vi "SWERVE_DRIVE_ACT.vi"(6 "Pass_Through_Time":dbl=-1.0 format="%33.4f", 8 "in Swerve Module States":T4[](array[typedef]) {"Angle"."SIN" format="%13.4f"; "Angle"."COS" format="%13.4f"; "Angle"."VALUE" format="%13.4f"}, 9 "Gyro_Heading_Rad":dbl, 10 "Swerve Drive Device Reference":T6[](array[typedef]), 11 "in SWERVE_DRIVE_KINEMATICS":T1 {"SavedModuleStates"."Angle"."SIN" format="%13.4f"; "SavedModuleStates"."Angle"."COS" format="%13.4f"; "SavedModuleStates"."Angle"."VALUE" format="%13.4f"; "PrevCoR"."Y" format="%14.3f"; "PrevCoR"."X" format="%14.3f"; "Modules"."Y" format="%14.3f"; "Modules"."X" format="%14.3f"}) -> (3 "out SWERVE_DRIVE_KINEMATICS":T1 {"SavedModuleStates"."Angle"."SIN" format="%13.4f"; "SavedModuleStates"."Angle"."COS" format="%13.4f"; "SavedModuleStates"."Angle"."VALUE" format="%13.4f"; "PrevCoR"."Y" format="%14.3f"; "PrevCoR"."X" format="%14.3f"; "Modules"."Y" format="%14.3f"; "Modules"."X" format="%14.3f"})   [LabVIEW 2019]
uses:
  <vilib>/Rock Robotics/WPI/ThirdParty/JAS_Junk/TrajLib/TypeDef/SWERVE_DRIVE_KINEMATICS.ctl
  <vilib>/Analysis/Matrix/Datatypes/RealMatrix.ctl
  <vilib>/Rock Robotics/WPI/ThirdParty/JAS_Junk/TrajLib/TypeDef/TRANSLATION2D.ctl
  <vilib>/Rock Robotics/WPI/ThirdParty/JAS_Junk/TrajLib/TypeDef/SWERVE_DRIVE_MODULE_STATE.ctl
  <vilib>/Rock Robotics/WPI/ThirdParty/JAS_Junk/TrajLib/TypeDef/ROTATION2D.ctl
  SWERVE_DRIVE_MODULE_TYPDEF.ctl
  <vilib>/Rock Robotics/WPI/MotorControl/WPI_MotorControlDeviceRef.ctl
  <vilib>/Rock Robotics/WPI/MotorControl/WPI_MotorControlType.ctl
  <vilib>/Rock Robotics/SystemInterfaces/DIO/FPGA_DIOPWMChannel.ctl
  <vilib>/Rock Robotics/WPI/PWM/WPI_PWMDeadband.ctl
  <vilib>/Rock Robotics/SystemInterfaces/DIO/FPGA_DIOChannel.ctl
  <vilib>/Rock Robotics/WPI/Encoder/WPI_EncoderDevRef.ctl
  <vilib>/Rock Robotics/SystemInterfaces/Encoder/FPGA_EncoderIdx.ctl
  <vilib>/Rock Robotics/SystemInterfaces/Counter/FPGA_CounterCtrSystemIndex.ctl
  <vilib>/Rock Robotics/WPI/Encoder/WPI_EncoderType.ctl
  <vilib>/Rock Robotics/WPI/ThirdParty/JAS_Junk/TrajLib/TypeDef/X_Y_PAIR.ctl
  <vilib>/Rock Robotics/WPI/ThirdParty/JAS_Junk/TrajLib/VI/Util_GetTime_U32.vi
  <vilib>/Rock Robotics/WPI/ThirdParty/JAS_Junk/TrajLib/MathUtil_InputModulus.vi
  <vilib>/Rock Robotics/WPI/ThirdParty/JAS_Junk/TrajLib/VI/FunctionGenerator_New.vi
  <vilib>/Rock Robotics/WPI/ThirdParty/JAS_Junk/TrajLib/VI/FunctionGenerator_Calculate.vi
  <vilib>/Rock Robotics/WPI/ThirdParty/JAS_Junk/TrajLib/PIDController_AtSetpoint.vi
  <vilib>/Rock Robotics/WPI/ThirdParty/JAS_Junk/TrajLib/PIDController_SetPIDF.vi
  <vilib>/Rock Robotics/WPI/ThirdParty/JAS_Junk/TrajLib/PIDController_SetDerivativeFilter.vi
  <vilib>/Rock Robotics/WPI/ThirdParty/JAS_Junk/TrajLib/PIDController_SetIntegratorRange.vi
  <vilib>/Rock Robotics/WPI/ThirdParty/JAS_Junk/TrajLib/PIDController_SetTolerancePandV.vi
  <vilib>/Rock Robotics/WPI/ThirdParty/JAS_Junk/TrajLib/PIDController_DisableContinousInput.vi
  <vilib>/Rock Robotics/WPI/ThirdParty/JAS_Junk/TrajLib/PIDController_EnableContinousInput.vi
  <vilib>/Rock Robotics/WPI/ThirdParty/JAS_Junk/TrajLib/PIDController_Reset.vi
  <vilib>/Rock Robotics/WPI/ThirdParty/JAS_Junk/TrajLib/PIDController_New.vi
  <vilib>/Rock Robotics/WPI/ThirdParty/JAS_Junk/TrajLib/PIDController_SetOutputLimits.vi
  <vilib>/Rock Robotics/WPI/ThirdParty/JAS_Junk/TrajLib/PIDController_NewPeriod.vi
  <vilib>/Rock Robotics/SystemInterfaces/NetworkCommunication/NetComm_UsageReport_report.vi
  SWERVE_DRIVE_GLOBALS.vi
  <vilib>/Rock Robotics/WPI/ThirdParty/JAS_Junk/TrajLib/VI/Util_GetTime_U64.vi
  <vilib>/gmath/interp.llb/Search Ordered Table.vi
  <vilib>/Rock Robotics/WPI/ThirdParty/JAS_Junk/TrajLib/Globals/Util_LibraryGlobals.vi
  <vilib>/Rock Robotics/WPI/ThirdParty/JAS_Junk/TrajLib/PIDController_AdvCalculate_FF_Sp_Pv.vi
  <vilib>/Rock Robotics/WPI/ThirdParty/JAS_Junk/TrajLib/Trajectory_Library.lvlib
  <vilib>/Analysis/Matrix/NI_Matrix.lvlib
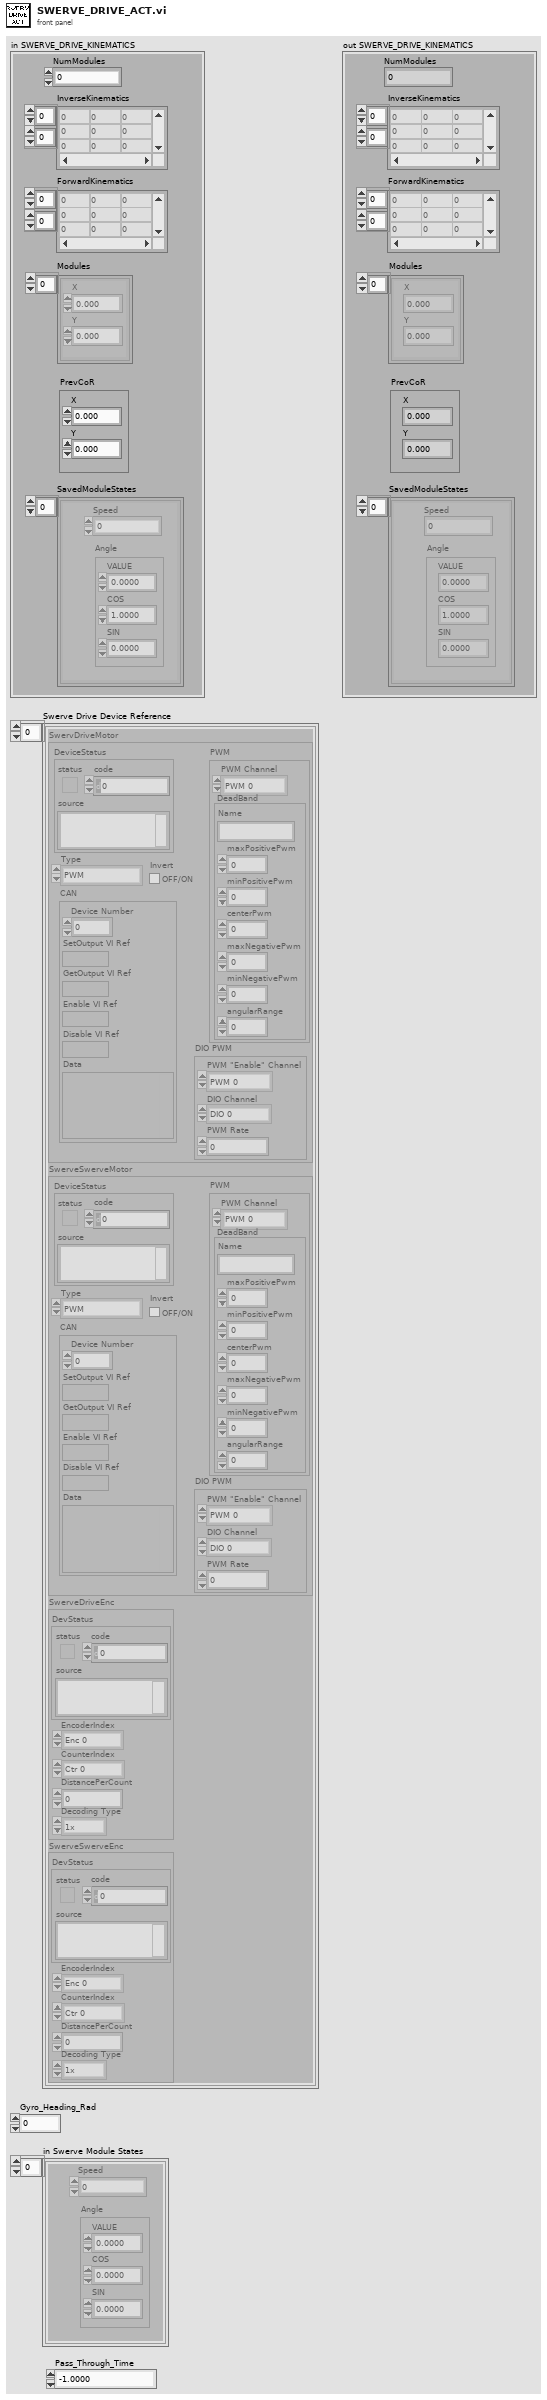
[diagram p1: front panel]
types:
  T1 = typedef "Trajectory_Library.lvlib/SWERVE_DRIVE_KINEMATICS.ctl" = cluster{"NumModules":i32, "InverseKinematics":T2, "ForwardKinematics":T2, "Modules":T3[], "PrevCoR":T3, "SavedModuleStates":T4[]}
  T2 = typedef "NI_Matrix.lvlib/RealMatrix.ctl" = dbl[][]
  T3 = typedef "Trajectory_Library.lvlib/TRANSLATION2D.ctl" = cluster{"X":dbl, "Y":dbl}
  T4 = typedef "Trajectory_Library.lvlib/SWERVE_DRIVE_MODULE_STATE.ctl" = cluster{"Speed":dbl, "Angle":T5}
  T5 = typedef "Trajectory_Library.lvlib/ROTATION2D.ctl" = cluster{"VALUE":dbl, "COS":dbl, "SIN":dbl}
  T6 = typedef "SWERVE_DRIVE_MODULE_TYPDEF.ctl" = cluster{"SwervDriveMotor":T7, "SwerveSwerveMotor":T7, "SwerveDriveEnc":T12, "SwerveSwerveEnc":T12}
  T7 = typedef "WPI_MotorControlDeviceRef.ctl" = cluster{"DeviceStatus":errorcluster, "Type":T8, "PWM":cluster{"PWM Channel":T9, "DeadBand":T10}, "CAN":cluster{"Device Number":u8, "SetOutput VI Ref":variant, "GetOutput VI Ref":variant, "Enable VI Ref":variant, "Disable VI Ref":variant, "Data":variant}, "Invert":bool, "DIO PWM":cluster{"PWM \"Enable\" Channel":T9, "DIOChannel":T11, "PWM Rate":dbl}}
  T8 = typedef "WPI_MotorControlType.ctl" = enum16{"PWM", "CAN", "DIO PWM"}
  T9 = typedef "FPGA_DIOPWMChannel.ctl" = enum8{"PWM 0", "PWM 1", "PWM 2", "PWM 3", "PWM 4", "PWM 5", "PWM 6", "PWM 7", "PWM 8", "PWM 9", "PWM MXP 0", "PWM MXP 1", "PWM MXP 2", "PWM MXP 3", "PWM MXP 4", "PWM MXP 5", "PWM MXP 6", "PWM MXP 7", "PWM MXP 8", "PWM MXP 9", "Invalid"}
  T10 = typedef "WPI_PWMDeadband.ctl" = cluster{"Name":string, "maxPositivePwm":i32, "minPositivePwm":i32, "centerPwm":i32, "maxNegativePwm":i32, "minNegativePwm":i32, "angularRange":u16}
  T11 = typedef "FPGA_DIOChannel.ctl" = enum8{"DIO 0", "DIO 1", "DIO 2", "DIO 3", "DIO 4", "DIO 5", "DIO 6", "DIO 7", "DIO 8", "DIO 9", "DIO MXP 0", "DIO MXP 1", "DIO MXP 2", "DIO MXP 3", "DIO MXP 4", "DIO MXP 5", "DIO MXP 6", "DIO MXP 7", "DIO MXP 8", "DIO MXP 9", "DIO MXP 10", "DIO MXP 11", "DIO MXP 12", "DIO MXP 13", "DIO MXP 14", "DIO MXP 15", "SPI Port CS1", "SPI Port CS2", "SPI Port CS3", "SPI Port MISO", "SPI Port MOSI", "Invalid"}
  T12 = typedef "WPI_EncoderDevRef.ctl" = cluster{"DevStatus":errorcluster, "EncoderIndex":T13, "CounterIndex":T14, "DistancePerCount":dbl, "Decoding Type":T15}
  T13 = typedef "FPGA_EncoderIdx.ctl" = enum8{"Enc 0", "Enc 1", "Enc 2", "Enc 3", "Enc 4", "Enc 5", "Enc 6", "Enc 7", "Invalid"}
  T14 = typedef "FPGA_CounterCtrSystemIndex.ctl" = enum8{"Ctr 0", "Ctr 1", "Ctr 2", "Ctr 3", "Ctr 4", "Ctr 5", "Ctr 6", "Ctr 7", "Invalid"}
  T15 = typedef "WPI_EncoderType.ctl" = enum16{"1x", "2x", "4x"}
  T16 = typedef "Trajectory_Library.lvlib/X_Y_PAIR.ctl" = cluster{"X":dbl, "Y":dbl}
  T17 = typedef "Trajectory_Library.lvlib/PID_ADV_LIMITS.ctl" = cluster{"MaxInput":dbl, "MinInput":dbl, "Continuous":bool, "MaxOutput":dbl, "MinOutput":dbl}
  T18 = typedef "Trajectory_Library.lvlib/PID_ADV_TUNING.ctl" = cluster{"Kf":dbl, "Kp":dbl, "Ki":dbl, "Kd":dbl, "MaximumIntegral":dbl, "MinimumIntegral":dbl, "Filter Derivative":bool}
  T19 = typedef "Trajectory_Library.lvlib/CHASSIS_SPEEDS.ctl" = cluster{"vX":dbl, "vY":dbl, "vOmega":dbl}
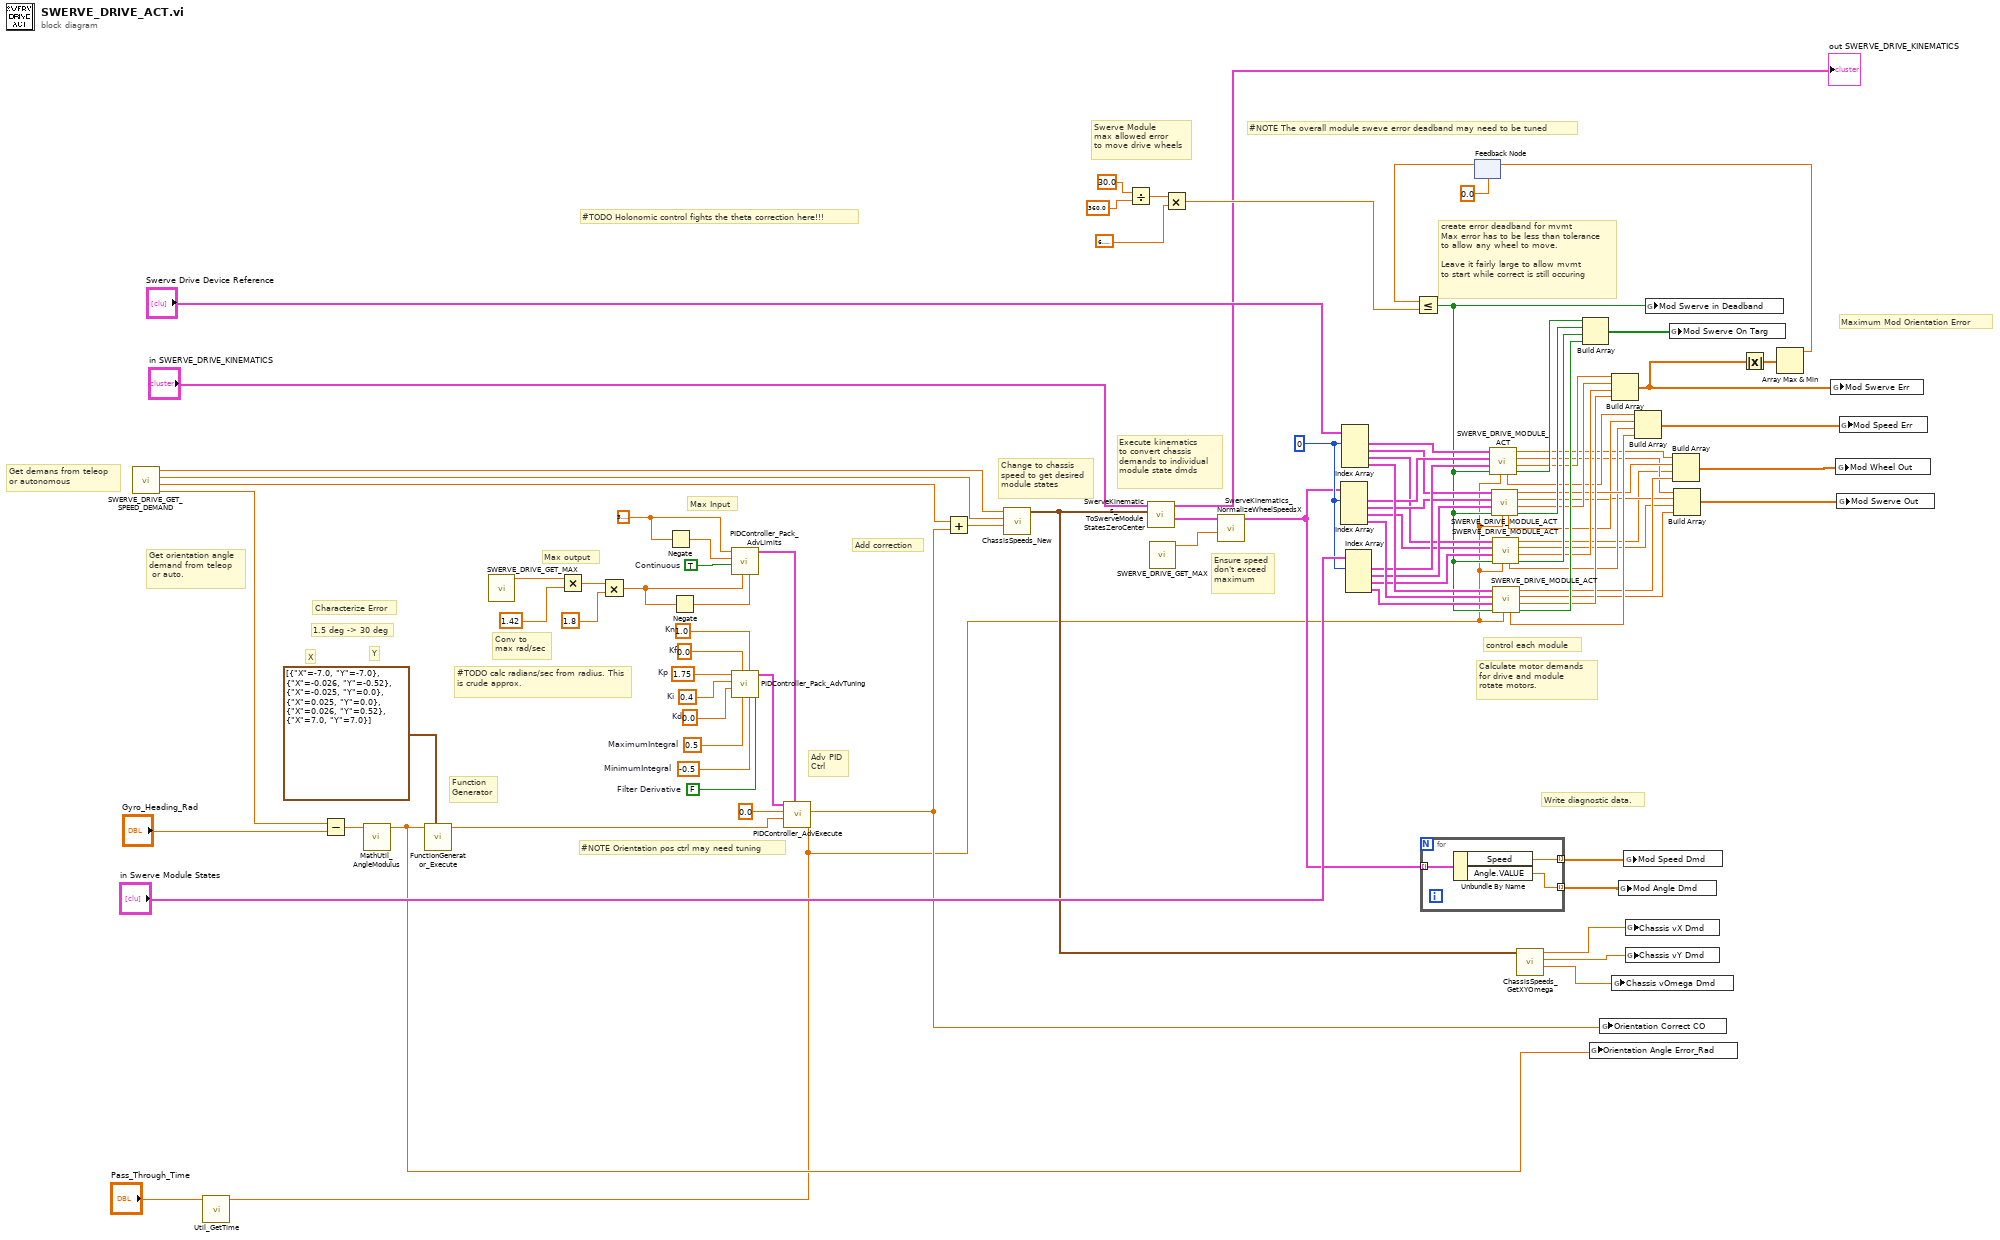
[diagram p0: block diagram]
diagram:
  w17 = 3.141592653589793
  w28 = 1.0  # Kn
  w27 = 1.75  # Kp
  w26 = 0.4  # Ki
  w25 = 0.0  # Kd
  w24 = 0.0  # Kf
  w23 = 0.5  # MaximumIntegral
  w22 = -0.5  # MinimumIntegral
  w21 = FALSE  # Filter Derivative
  w20 = TRUE  # Continuous
  w64 = 0 ("index")
  # "Swerve Module\nmax allowed error\nto move drive wheels"
  # "Characterize Error"
  # "Conv to\nmax rad/sec"
  # "Max output"
  # "Max Input"
  # "Adv PID\nCtrl"
  # "1.5 deg -> 30 deg"
  # "Function\nGenerator"
  # "Y"
  # "X"
  # "Ensure speed\ndon't exceed\nmaximum"
  # "Write diagnostic data."
  # "Maximum Mod Orientation Error"
  # "#NOTE The overall module sweve error deadband may need to be tuned"
  # "create error deadband for mvmt\nMax error has to be less than tolerance\nto allow any wheel to move. \n\nLeave it fairly large to allow mvmt\nto start while correct is still occuring"
  # "#TODO Holonomic control fights the theta correction here!!!"
  # "Calculate motor demands\nfor drive and module \nrotate motors."
  # "Execute kinematics\nto convert chassis \ndemands to individual\nmodule state dmds"
  # "Get orientation angle\ndemand from teleop\n or auto."
  # "Add correction"
  # "Get demans from teleop\nor autonomous"
  # "#TODO calc radians/sec from radius. This is crude approx."
  # "#NOTE Orientation pos ctrl may need tuning"
  # "control each module"
  # "Change to chassis \nspeed to get desired\nmodule states"
  n1 = call "SWERVE_DRIVE_GET_SPEED_DEMAND.vi"() -> ("Drv Rotation Orentation Dmd"=w9:dbl, "Drv Angular Vel Dmd"=w42:dbl, "Drv Y Vel Dmd"=w43:dbl, "Drv X Vel Dmd"=w44:dbl)  [unwired: 8 in]
  n2 = call <vilib>:"Util_GetTime.vi"("Pass_Through_Time"="Pass_Through_Time") -> ("FPGA_Time_Seconds"=w1:dbl)  [unwired: 8 in, 2 out]
  n3 = Subtract(x=w9, y="Gyro_Heading_Rad") -> (x-y=w4:dbl)
  n4 = call <vilib>:"MathUtil_AngleModulus.vi"("InputAngle"=w4) -> ("ModulsAngle"=w2:dbl)  [unwired: 10 in]
  n5 = call <vilib>:"FunctionGenerator_Execute.vi"("X Y Pairs"=T16[] [{"X"=-7.0, "Y"=-7.0}, {"X"=-0.026, "Y"=-0.52}, {"X"=-0.025, "Y"=0.0}, {"X"=0.025, "Y"=0.0}, {"X"=0.026, "Y"=0.52}, {"X"=7.0, "Y"=7.0}], "Input Value"=w2) -> ("Output Value"=w3:dbl)  [unwired: 9 in]
  n6 = call "SWERVE_DRIVE_GET_MAX.vi"() -> ("Max Wheel Vel (Meter/Sec)"=w14:dbl)  [unwired: 10 in, 1 out]
  n7 = Multiply(x=w14, y=1.42) -> (x*y=w13:dbl)
  n8 = Multiply(x=w13, y=1.8) -> (x*y=w10:dbl)
  n9 = Negate(x=w17) -> (-x=w16:dbl)
  n10 = Negate(x=w10) -> (-x=w11:dbl)
  n11 = call <vilib>:"PIDController_Pack_AdvLimits.vi"("MinOutput"=w11, "MaxOutput"=w10, "Continuous"=w20, "MinInput"=w16, "MaxInput"=w17) -> ("Adv PID Limits"=w18:T17)  [unwired: 6 in]
  n12 = call <vilib>:"PIDController_Pack_AdvTuning.vi"("Filter Derivative"=w21, "MinimumIntegral"=w22, "Kn"=w28, "MaximumIntegral"=w23, "Kf"=w24, "Kd"=w25, "Ki"=w26, "Kp"=w27) -> ("Adv PID Tuning"=w19:T18)  [unwired: 3 in]
  n13 = call <vilib>:"PIDController_AdvExecute.vi"("Time"=w1, "Adv PID Limits"=w18, "SP-SetPoint"=w3, "PV-Measurement"=0.0, "Adv PID Tuning"=w19) -> ("CO-ControlOutput"=w5:dbl)  [unwired: 4 in, 2 out]
  n14 = Add(x=w42, y=w5) -> (x+y=w65:dbl)
  n15 = call <vilib>:"ChassisSpeeds_New.vi"("vAngular"=w65, "vY"=w43, "vX"=w44) -> ("CHASSIS"=w41:T19)  [unwired: 8 in]
  n16 = Divide(x=30.0, y=360.0) -> (x/y=w90:dbl)
  n17 = call <vilib>:"SwerveKinematics_ToSwerveModuleStatesZeroCenter.vi"("ChassisSpeeds"=w41, "in SWERVE_DRIVE_KINEMATICS"="in SWERVE_DRIVE_KINEMATICS") -> ("ModuleStates"=w45:T4[], "out SWERVE_DRIVE_KINEMATICS"=→"out SWERVE_DRIVE_KINEMATICS":T1)  [unwired: 8 in]
  n18 = call "SWERVE_DRIVE_GET_MAX.vi"() -> ("Max Wheel Vel (Meter/Sec)"=w47:dbl)  [unwired: 10 in, 1 out]
  n19 = Multiply(x=w90, y=6.283185307179586) -> (x*y=w94:dbl)
  n20 = call <vilib>:"SwerveKinematics_NormalizeWheelSpeedsX.vi"("AttainableMaxSpeed"=w47, "in WheelStates"=w45) -> ("out WheelStates"=w52:T4[])  [unwired: 9 in]
  n21 = Index Array(array=w52, index #1=w64) -> (element #1=w53:T4, element #2=w54:T4, element #3=w55:T4, element #4=w69:T4)  [unwired: 3 in]
  n22 = Index Array(array="Swerve Drive Device Reference", index #1=w64) -> (element #1=w49:T6, element #2=w50:T6, element #3=w51:T6, element #4=w68:T6)  [unwired: 3 in]
  n23 = Index Array(array="in Swerve Module States", index #1=w64) -> (element #1=w56:T4, element #2=w57:T4, element #3=w58:T4, element #4=w70:T4)  [unwired: 3 in]
  n24 = for {
    tunnel: w52 -> [w97] mode=indexing
    tunnel: [w96] -> w39 mode=indexing
    tunnel: [w95] -> w40 mode=indexing
    n25 = Unbundle By Name(w97) -> ("Speed"=w95:dbl, "Angle.VALUE"=w96:dbl)
  }
  n26 = feedback #1(0.0) -> (w87:dbl)
  n27 = Less Or Equal?(x=w87, y=w94) -> (x <= y?=w31:bool)
  n28 = call "SWERVE_DRIVE_MODULE_ACT.vi"("Pass_Through_Time"=w1, "SwervePosInDeadband"=w31, "Swerve Sense"=w56, "Swerve Dmd"=w53, "Swerve Module TypDef"=w49) -> ("SwerveOnTarget"=w80:bool, "SwervePosError"=w75:dbl, "Swerve Motor Dmd"=w61:dbl, "Wheel Motor Dmd"=w59:dbl, "WheelSpeedErr"=w71:dbl)  [unwired: 2 in]
  n29 = call "SWERVE_DRIVE_MODULE_ACT.vi"("Pass_Through_Time"=w1, "SwervePosInDeadband"=w31, "Swerve Sense"=w57, "Swerve Dmd"=w54, "Swerve Module TypDef"=w50) -> ("SwerveOnTarget"=w81:bool, "SwervePosError"=w76:dbl, "Swerve Motor Dmd"=w62:dbl, "Wheel Motor Dmd"=w74:dbl, "WheelSpeedErr"=w72:dbl)  [unwired: 2 in]
  n30 = call "SWERVE_DRIVE_MODULE_ACT.vi"("Pass_Through_Time"=w1, "SwervePosInDeadband"=w31, "Swerve Sense"=w58, "Swerve Dmd"=w55, "Swerve Module TypDef"=w51) -> ("SwerveOnTarget"=w82:bool, "SwervePosError"=w77:dbl, "Swerve Motor Dmd"=w63:dbl, "Wheel Motor Dmd"=w60:dbl, "WheelSpeedErr"=w73:dbl)  [unwired: 2 in]
  n31 = call "SWERVE_DRIVE_MODULE_ACT.vi"("Pass_Through_Time"=w1, "SwervePosInDeadband"=w31, "Swerve Sense"=w70, "Swerve Dmd"=w69, "Swerve Module TypDef"=w68) -> ("SwerveOnTarget"=w83:bool, "SwervePosError"=w78:dbl, "Swerve Motor Dmd"=w67:dbl, "Wheel Motor Dmd"=w66:dbl, "WheelSpeedErr"=w79:dbl)  [unwired: 2 in]
  n32 = call <vilib>:"ChassisSpeeds_GetXYOmega.vi"("CHASSIS"=w41) -> ("vAngular"=w36:dbl, "vY"=w37:dbl, "vX"=w38:dbl)  [unwired: 8 in]
  n33 = Build Array(w80, w81, w82, w83) -> (w30:bool[])
  n34 = global write "SWERVE_DRIVE_GLOBALS.vi" "Orientation Angle Error_Rad"(w2) -> ()
  n35 = global write "SWERVE_DRIVE_GLOBALS.vi" "Orientation Correct CO"(w5) -> ()
  n36 = Build Array(w75, w76, w77, w78) -> (w33:dbl[])
  n37 = global write "SWERVE_DRIVE_GLOBALS.vi" "Chassis vOmega Dmd"(w36) -> ()
  n38 = global write "SWERVE_DRIVE_GLOBALS.vi" "Mod Angle Dmd"(w39) -> ()
  n39 = global write "SWERVE_DRIVE_GLOBALS.vi" "Mod Speed Dmd"(w40) -> ()
  n40 = global write "SWERVE_DRIVE_GLOBALS.vi" "Chassis vX Dmd"(w38) -> ()
  n41 = global write "SWERVE_DRIVE_GLOBALS.vi" "Chassis vY Dmd"(w37) -> ()
  n42 = Build Array(w71, w72, w73, w79) -> (w32:dbl[])
  n43 = global write "SWERVE_DRIVE_GLOBALS.vi" "Mod Swerve in Deadband"(w31) -> ()
  n44 = global write "SWERVE_DRIVE_GLOBALS.vi" "Mod Swerve On Targ"(w30) -> ()
  n45 = Build Array(w59, w74, w60, w66) -> (w35:dbl[])
  n46 = Build Array(w61, w62, w63, w67) -> (w34:dbl[])
  n47 = Absolute Value(x=w33) -> (abs(x)=w84:dbl[])
  n48 = Array Max & Min(array=w84) -> (max value=w85:dbl)  [unwired: 3 out]
  n49 = feedback-in #1(w85) -> ()
  n50 = global write "SWERVE_DRIVE_GLOBALS.vi" "Mod Swerve Err"(w33) -> ()
  n51 = global write "SWERVE_DRIVE_GLOBALS.vi" "Mod Wheel Out"(w35) -> ()
  n52 = global write "SWERVE_DRIVE_GLOBALS.vi" "Mod Swerve Out"(w34) -> ()
  n53 = global write "SWERVE_DRIVE_GLOBALS.vi" "Mod Speed Err"(w32) -> ()
